vi "SPI_Test.vi"() -> ()   [LabVIEW 2012]
uses:
  <vilib>/rvi/eio/common/nirviEmuTemplateMethod_errors.vi
  <vilib>/eio/EIONode/EIONode.xnode
panel:
  out "Power":bool
  in  "Power":bool
  out "MISO":bool
  in  "MISO":bool
  out "MOSI":bool
  in  "MOSI":bool
  out "SCK":bool
  in  "SCK":bool
  in  "stop":bool
  in  "SS":bool
  out "SS":bool
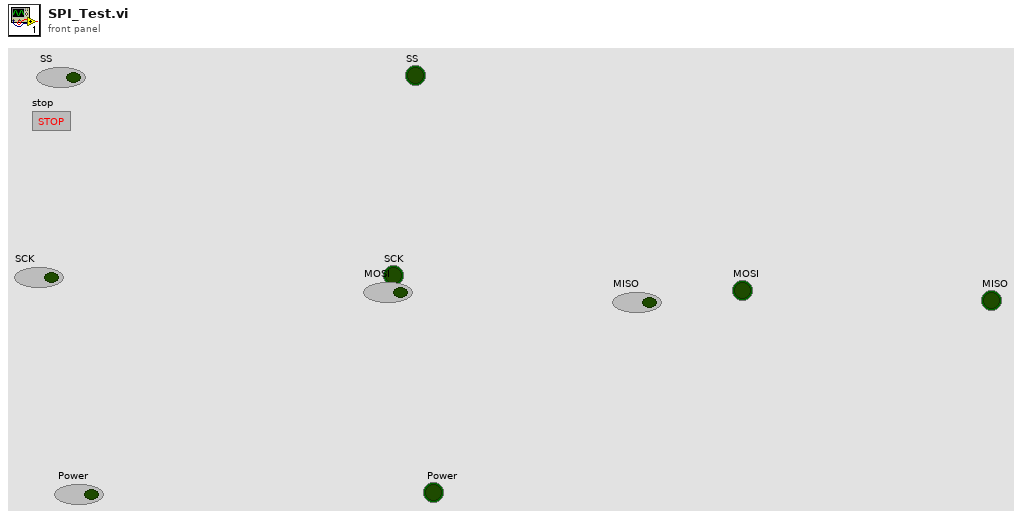
[diagram p1: front panel]
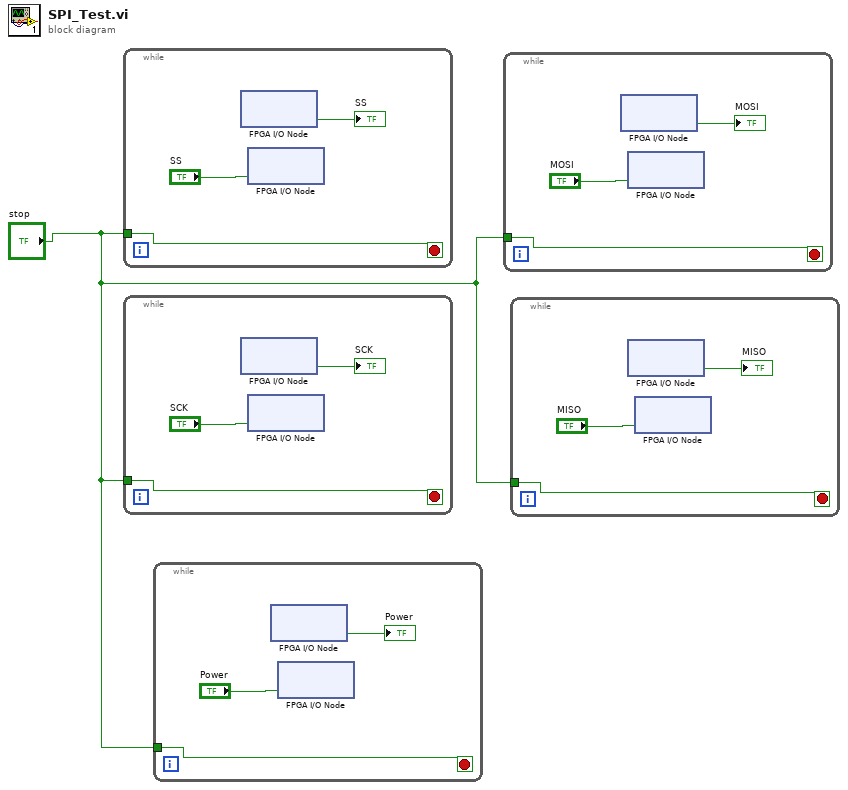
[diagram p0: block diagram]
diagram:
  n1 = while {
    tunnel: "stop" -> [w2]
    stop <- w2 stop-if-true
    n2 = xnode "FPGA I/O Node"() -> ("DIO5"=→"SS":bool)  [unwired: 1 in, 1 out]
    n3 = xnode "FPGA I/O Node"("DIO5"="SS") -> ()  [unwired: 1 in, 1 out]
  }
  n4 = while {
    tunnel: "stop" -> [w5]
    stop <- w5 stop-if-true
    n5 = xnode "FPGA I/O Node"() -> ("DIO6"=→"SCK":bool)  [unwired: 1 in, 1 out]
    n6 = xnode "FPGA I/O Node"("DIO6"="SCK") -> ()  [unwired: 1 in, 1 out]
  }
  n7 = while {
    tunnel: "stop" -> [w8]
    stop <- w8 stop-if-true
    n8 = xnode "FPGA I/O Node"() -> ("DIO4"=→"Power":bool)  [unwired: 1 in, 1 out]
    n9 = xnode "FPGA I/O Node"("DIO4"="Power") -> ()  [unwired: 1 in, 1 out]
  }
  n10 = while {
    tunnel: "stop" -> [w11]
    stop <- w11 stop-if-true
    n11 = xnode "FPGA I/O Node"() -> ("DIO7"=→"MOSI":bool)  [unwired: 1 in, 1 out]
    n12 = xnode "FPGA I/O Node"("DIO7"="MOSI") -> ()  [unwired: 1 in, 1 out]
  }
  n13 = while {
    tunnel: "stop" -> [w14]
    stop <- w14 stop-if-true
    n14 = xnode "FPGA I/O Node"() -> ("DIO8"=→"MISO":bool)  [unwired: 1 in, 1 out]
    n15 = xnode "FPGA I/O Node"("DIO8"="MISO") -> ()  [unwired: 1 in, 1 out]
  }
